vi "GetFormatTags.vi"(8 "error in (no error)":errorcluster, 11 "Format String":string) -> (0 "error out":errorcluster, 3 "Format Tags":map{string, string}(c390))   [LabVIEW 2019, in "LabErrorUX.lvclass"]
uses:
  LabErrorUX.lvclass
  LabErrorUX.lvclass/LabErrorUX.ctl
  <vilib>/SLL Toolkit/SLL String/SLL String.lvlib
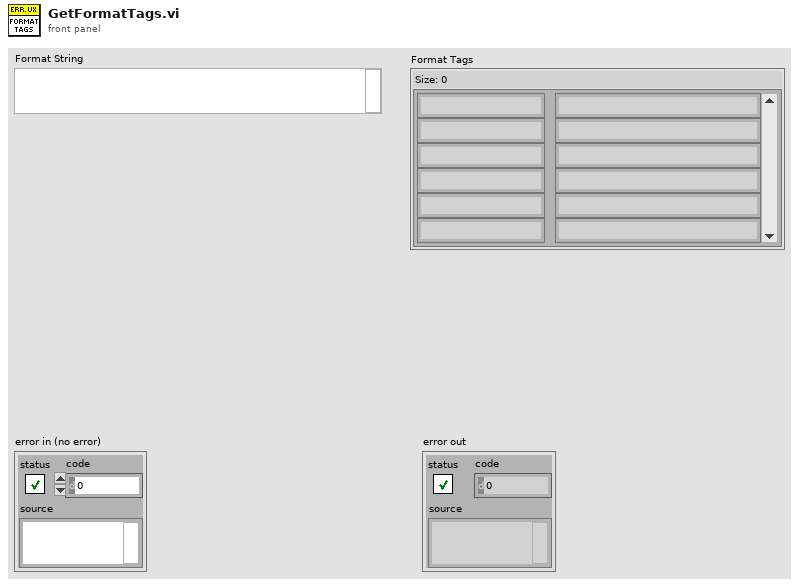
[diagram p1: front panel]
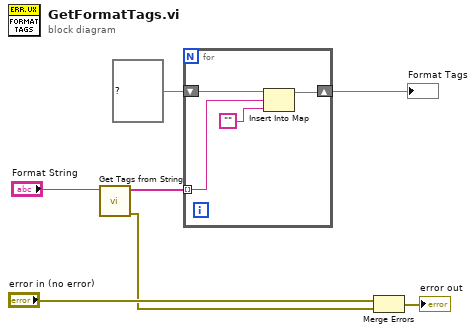
[diagram p0: block diagram]
diagram:
  n1 = call <vilib>:"Get Tags from String.vi"("Input String"="Format String") -> ("error out"=w2:errorcluster, "Tags[]"=w5:string[])  [unwired: 9 in]
  n2 = for {
    shift-right: [w10] -> w4
    shift-left: map{string, string} {} ("Format Tags") -> [w11]
    tunnel: w5 -> [w9] mode=indexing
    n3 = Insert Into Map(map in=w11, key=w9, value="") -> (map out=w10:map{string, string})  [unwired: 2 out]
  }
  "Format Tags" <- w4
  n4 = Merge Errors("error in (no error)", w2) -> (→"error out":errorcluster)
